vi "Memory.Pointer.Move Block (safe).vi"(0 "src Pointer in":refnum<class "Memory.Pointer.lvclass">, 1 "length":i64 format="%d bytes", 5 "dst Pointer in":refnum<class "Memory.Pointer.lvclass">, 7 "src offset (0)":i64 format="%d bytes", 9 "dst offset (0)":i64 format="%d bytes", 11 "error in (no error)":errorcluster) -> (4 "src Pointer out":refnum<class "Memory.Pointer.lvclass">, 6 "dst Pointer out":refnum<class "Memory.Pointer.lvclass">, 15 "error out":errorcluster)   [LabVIEW 2016, in "LabVIEW Memory Manager.lvlib" / "Memory.Pointer.lvclass"]
uses:
  Memory.Pointer.lvclass
  Memory.Pointer.lvclass/Memory.Pointer.ctl
  Accessors/Memory.Pointer.Get Size.vi
  Memory.Pointer.Bounds Check.Length.vi
  Accessors/Memory.Pointer.Get Address.vi
  VIs/Memory.Truncate I64 to I32.vi
  LabVIEW Memory Manager.lvlib
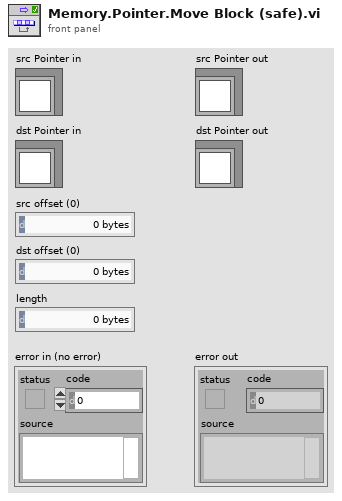
[diagram p1: front panel]
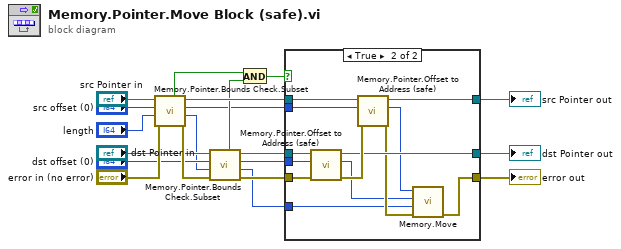
[diagram p0: block diagram]
diagram:
  n1 = call "Memory.Pointer.Bounds Check.Subset.vi"("error in (no error)"="error in (no error)", "length"="length", "offset"="src offset (0)", "Pointer in"="src Pointer in") -> ("error out"=w20:errorcluster, "length out"=w3:i64, "offset out"=w4:i64, "Pointer out"=w14:refnum<class "Memory.Pointer.lvclass">, "subset valid"=w10:bool)  [unwired: 3 in]
  n2 = call "Memory.Pointer.Bounds Check.Subset.vi"("error in (no error)"=w20, "length"=w3, "offset"="dst offset (0)", "Pointer in"="dst Pointer in") -> ("error out"=w11:errorcluster, "length out"=w2:i64, "offset out"=w5:i64, "Pointer out"=w15:refnum<class "Memory.Pointer.lvclass">, "subset valid"=w9:bool)  [unwired: 3 in]
  n3 = And(x=w10, y=w9) -> (x .and. y?=w16:bool)
  n4 = case shown="True" w16 {
    tunnel: w15 -> [w23 w34]
    tunnel: w14 -> [w21 w35]
    tunnel: [w23 w31] -> w12
    tunnel: [w21 w30] -> w13
    tunnel: w11 -> [w22 w33]
    tunnel: w5 -> [_ w32]
    tunnel: w4 -> [_ w29]
    tunnel: w2 -> [_ w24]
    tunnel: [w22 w27] -> w1
    frame False {
      # "#TODO\nThrow error."
    }
    frame True {
      n5 = call "Memory.Pointer.Offset to Address (safe).vi"("error in (no error)"=w33, "offset"=w32, "Pointer in"=w34) -> ("error out"=w36:errorcluster, "address"=w25:u64, "Pointer out"=w31:refnum<class "Memory.Pointer.lvclass">)  [unwired: 5 in, 1 out]
      n6 = call "Memory.Pointer.Offset to Address (safe).vi"("error in (no error)"=w36, "offset"=w29, "Pointer in"=w35) -> ("error out"=w28:errorcluster, "address"=w26:u64, "Pointer out"=w30:refnum<class "Memory.Pointer.lvclass">)  [unwired: 5 in, 1 out]
      n7 = call "Memory.Move.vi"("error in (no error)"=w28, "size"=w24, "dst address"=w25, "src address"=w26) -> ("error out"=w27:errorcluster)  [unwired: 7 in]
    }
  }
  "error out" <- w1
  "src Pointer out" <- w13
  "dst Pointer out" <- w12
